vi "Other VI with event.vi"() -> ()   [LabVIEW 2011]
uses:
  Event FGV Actions.ctl
panel:
  in  "event data (any text)":string="FGV Event"
  in  "Other VI Event":bool
  out "error out":errorcluster
  in  "error in (no error)":errorcluster
  in  "stop":bool
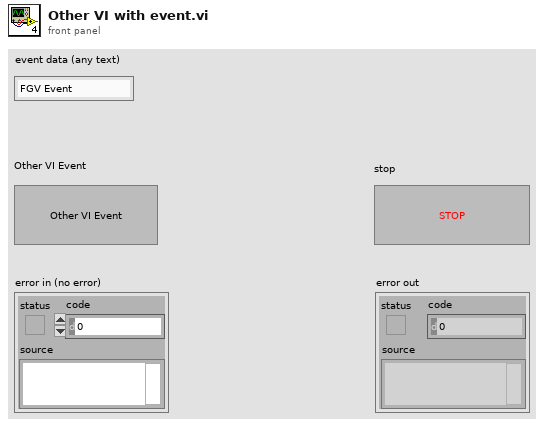
[diagram p1: front panel]
types:
  T1 = typedef "Event FGV Actions.ctl" = enum16{"Register Event", "Fire Event"}
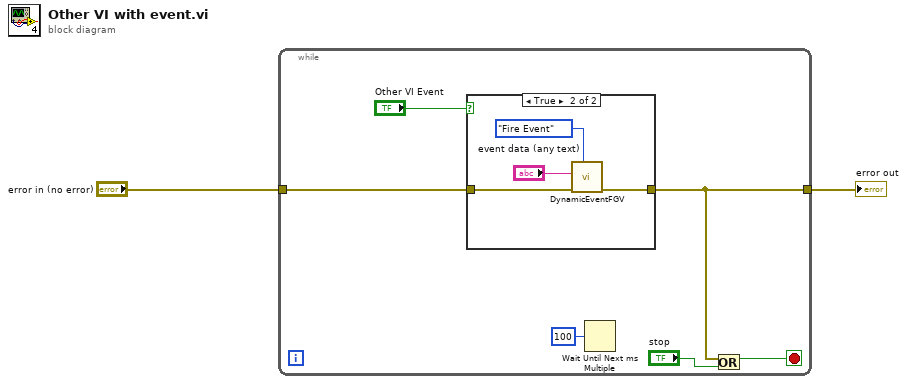
[diagram p0: block diagram]
diagram:
  n1 = while {
    tunnel: "error in (no error)" -> [w7]
    tunnel: [w3] -> w2
    stop <- w4 stop-if-true
    n2 = case shown="True" "Other VI Event" {
      tunnel: w7 -> [w9 w12]
      tunnel: [w9 w13] -> w3
      frame False {
      }
      frame True {
        n3 = call "DynamicEventFGV.vi"("Event FGV Actions"=Event_FGV_Actions."Fire Event", "error in (no error)"=w12, "event data"="event data (any text)") -> ("error out"=w13:errorcluster)  [unwired: 6 in, 2 out]
      }
    }
    n4 = Wait Until Next ms Multiple(millisecond multiple=u32 100) -> ()  [unwired: 1 out]
    n5 = Or(x=w3, y="stop") -> (x .or. y?=w4:bool)
  }
  "error out" <- w2
